vi "Untitled 1.vi"() -> ()   [LabVIEW 2013]
uses:
  <vilib>/Instr/_visa.llb/VISA Configure Serial Port (Instr).vi
panel:
  out "Temperatura":cluster{dbl, dbl, "Setpoint temperatura":u8}(graph)
  out "close door":string="cerrada"
  out "open door":string="abierta"
  in  "Setpoint temperatura":u8(knob)=25 scale=0.0..100.0
  in  "?":bool
  in  "stop":bool
  in  "VISA resource name":refnum<visa-resource-name>
  # "electroválvula"
  # "abrir"
  # "cerrar"
  # "Compuerta:"
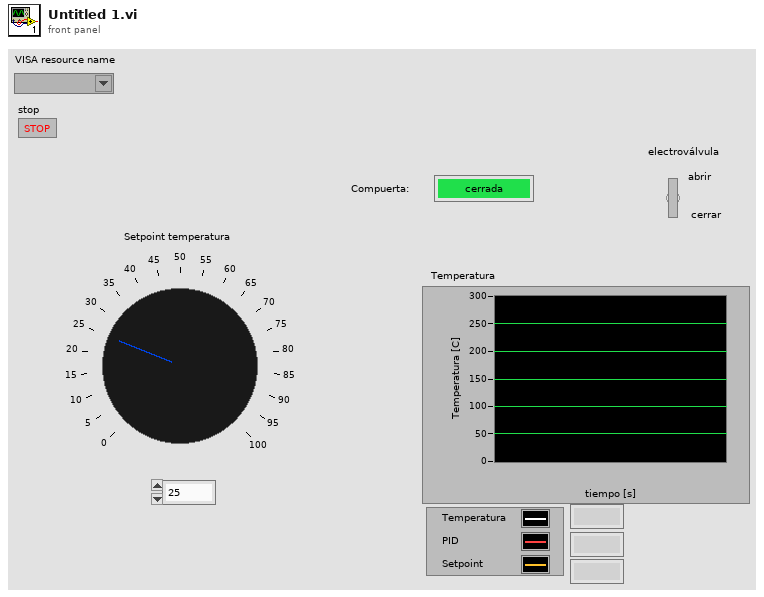
[diagram p1: front panel]
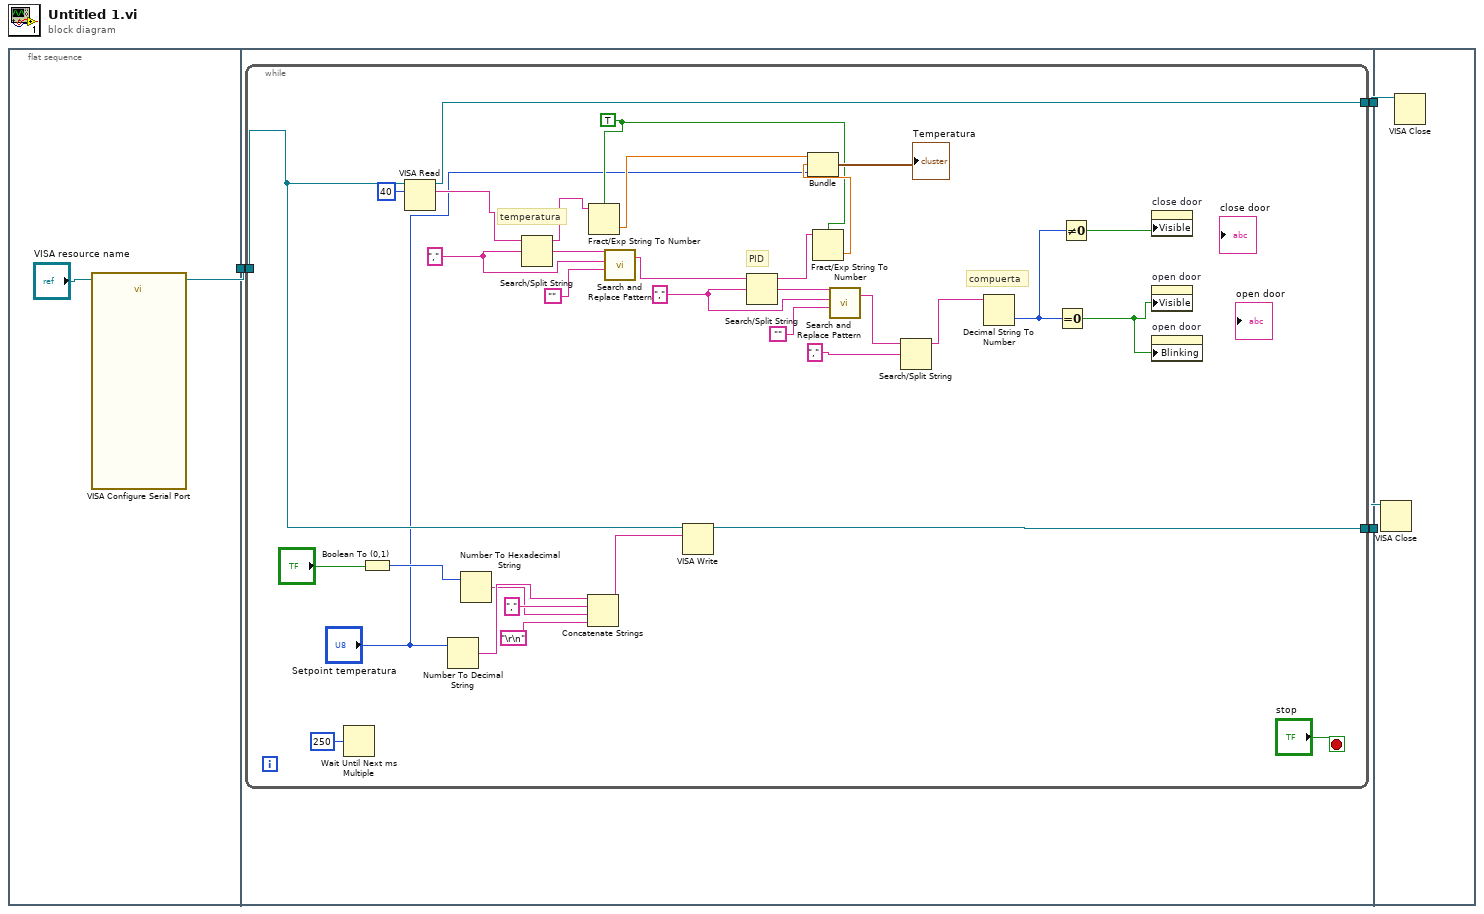
[diagram p0: block diagram]
diagram:
  n1 = flat-sequence {
    tunnel: [w4] -> w3
    tunnel: w3 -> [w8]
    tunnel: [w7] -> w2
    tunnel: [w6] -> w1
    tunnel: w2 -> [w44]
    tunnel: w1 -> [w43]
    frame #0 {
      n2 = call-poly "VISA Configure Serial Port"("VISA resource name"="VISA resource name") -> ("VISA resource name out"=w4:refnum<visa-resource-name>)  [unwired: 13 in, 1 out]
    }
    frame #1 {
      n3 = while {
        tunnel: w8 -> [w40]
        tunnel: [w39] -> w7
        tunnel: [w35] -> w6
        stop <- "stop" stop-if-true
        w10 = TRUE
        w29 = "," ("search string/char (-)")
        w32 = "," ("search string/char (-)")
        # "compuerta"
        # "PID"
        # "temperatura"
        n4 = Wait Until Next ms Multiple(millisecond multiple=u32 250) -> ()  [unwired: 1 out]
        n5 = Boolean To (0,1)(Boolean="?") -> (0, 1=w37:i16)
        n6 = VISA Read(VISA resource name=w40, byte count=u32 40) -> (VISA resource name out=w35:refnum<visa-resource-name>, read buffer=w34:string)  [unwired: 1 in, 2 out]
        n7 = Number To Decimal String(number="Setpoint temperatura") -> (decimal integer string=w22:string)  [unwired: 1 in]
        n8 = Number To Hexadecimal String(2:w37) -> (0:w21:string)  [unwired: 1 in]
        n9 = Search/Split String(string=w34, search string/char (-)=w32) -> (substring before match=w14:string, match + rest of string=w33:string)  [unwired: 1 in, 1 out]
        n10 = Concatenate Strings(w22, "," ("string"), w21, "\r\n") -> (w25:string)
        n11 = Fract/Exp String To Number(use system decimal point (T)=w10, string=w14) -> (number=w13:dbl)  [unwired: 2 in, 1 out]
        n12 = call <vilib>:"Search and Replace Pattern.vi"("string"=w33, "regular expression (\"\")"=w32, "replace string (\"\")"="") -> ("result string"=w28:string)  [unwired: 2 in, 1 out]
        n13 = VISA Write(VISA resource name=w40, write buffer=w25) -> (VISA resource name out=w39:refnum<visa-resource-name>)  [unwired: 1 in, 2 out]
        n14 = Search/Split String(string=w28, search string/char (-)=w29) -> (substring before match=w12:string, match + rest of string=w30:string)  [unwired: 1 in, 1 out]
        n15 = Fract/Exp String To Number(use system decimal point (T)=w10, string=w12) -> (number=w11:dbl)  [unwired: 2 in, 1 out]
        n16 = Bundle(w13, w11, "Setpoint temperatura"="Setpoint temperatura") -> (→"Temperatura":cluster{dbl, dbl, "Setpoint temperatura":u8})  [unwired: 1 in]
        n17 = call <vilib>:"Search and Replace Pattern.vi"("string"=w30, "regular expression (\"\")"=w29, "replace string (\"\")"="") -> ("result string"=w26:string)  [unwired: 2 in, 1 out]
        n18 = Search/Split String(string=w26, search string/char (-)=",") -> (substring before match=w19:string)  [unwired: 1 in, 2 out]
        n19 = Decimal String To Number(string=w19) -> (number=w16:i32)  [unwired: 2 in, 1 out]
        n20 = Equal To 0?(x=w16) -> (x = 0?=w18:bool)
        n21 = Not Equal To 0?(x=w16) -> (x != 0?=w17:bool)
        n22 = property on="close door" class="Str"("Visible"=w17) -> ()  [unwired: 2 in, 2 out]
        n23 = property on="open door" class="Str"("Visible"=w18) -> ()  [unwired: 2 in, 2 out]
        n24 = property on="open door" class="Str"("Blinking"=w18) -> ()  [unwired: 2 in, 2 out]
      }
    }
    frame #2 {
      n25 = VISA Close(VISA resource name=w44) -> ()  [unwired: 1 in, 1 out]
      n26 = VISA Close(VISA resource name=w43) -> ()  [unwired: 1 in, 1 out]
    }
  }
